vi "Eliminated.vi"(6 "Column":i32, 8 "Row":i32, 9 "Killer":i32, 10 "Team":i32, 11 "Great Wall in":refnum<class "Great Wall.lvclass">) -> (3 "Great Wall out":refnum<class "Great Wall.lvclass">)   [LabVIEW 2020, in "Great Wall.lvclass"]
uses:
  Great Wall.lvclass
  Great Wall.lvclass/Great Wall.ctl
  Square/Square.lvclass
  DS Square Library/DS Square.lvlib
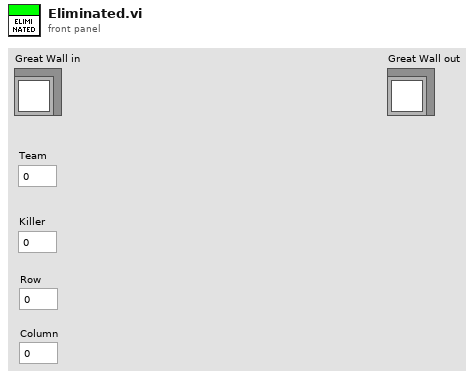
[diagram p1: front panel]
types:
  T1 = typedef "Common.lvlib/Position.ctl" = cluster{"Column":i32, "Row":i32}
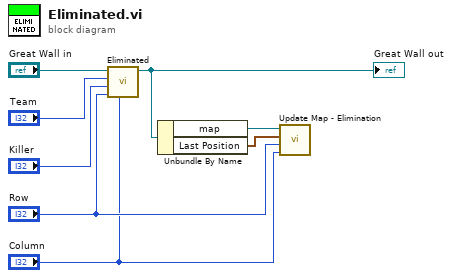
[diagram p0: block diagram]
diagram:
  n1 = call-parent "Eliminated.vi"("Column"="Column", "Row"="Row", "Killer Index"="Killer", "Team Index"="Team", "Square in"="Great Wall in") -> ("Square out"=w5:refnum<class "Great Wall.lvclass">)  [unwired: 6 in]
  "Great Wall out" <- w5
  n2 = Unbundle By Name(w5) -> ("map"=w4:refnum<data-value>, "Last Position"=w3:T1)
  n3 = call "Update Map - Elimination.vi"("Column"="Column", "Row"="Row", "Last Position"=w3, "map in"=w4) -> ()  [unwired: 7 in, 1 out]
